vi "RGB to Color I2C.vi"(6 "B":u8, 7 "G":u8, 8 "R":u8) -> (0 "LEDout":i32[](array[numeric]), 1 "Blue Color":i32[](array[numeric]), 2 "Green Color":i32[](array[numeric]), 3 "Red Color":i32[](array[numeric]), 4 "Color":u32(colorbox))   [LabVIEW 2012]
doc: "Converts a red, green, and blue value from 0 to 255 to the corresponding RGB color."
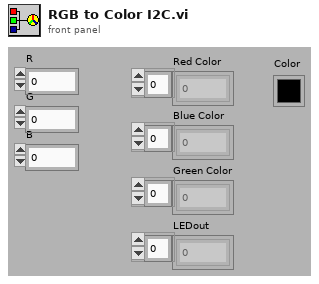
[diagram p1: front panel]
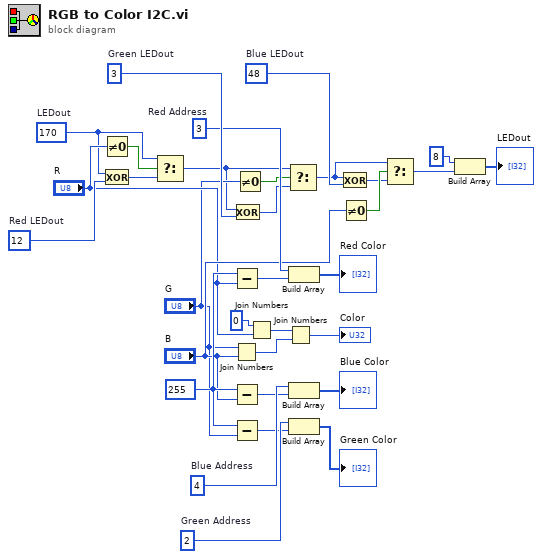
[diagram p0: block diagram]
diagram:
  w14 = 170  # LEDout
  w22 = 4  # Blue Address
  w16 = 2  # Green Address
  w24 = 3  # Red Address
  w25 = 48  # Blue LEDout
  w26 = 3  # Green LEDout
  w27 = 12  # Red LEDout
  w32 = 255
  n1 = Not Equal To 0?(x="R") -> (x != 0?=w15:bool)
  n2 = Exclusive Or(1:w27, 2:w14) -> (0:w13:i32)
  n3 = Select(t=w14, s=w15, f=w13) -> (s? t:f=w11:i32)
  n4 = Subtract(x=w32, y="R") -> (x-y=w3:i32)
  n5 = Join Numbers(hi="G", lo="B") -> ((hi.lo)=w29:u16)
  n6 = Subtract(x=w32, y="B") -> (x-y=w1:i32)
  n7 = Subtract(x=w32, y="G") -> (x-y=w2:i32)
  n8 = Exclusive Or(1:w26, 2:w11) -> (0:w10:i32)
  n9 = Not Equal To 0?(x="G") -> (x != 0?=w12:bool)
  n10 = Join Numbers(hi=u8 0, lo="R") -> ((hi.lo)=w30:u16)
  n11 = Join Numbers(hi=w30, lo=w29) -> ((hi.lo)=→"Color":u32)
  n12 = Select(t=w11, s=w12, f=w10) -> (s? t:f=w4:i32)
  n13 = Build Array(w24, w3) -> (→"Red Color":i32[])
  n14 = Build Array(w22, w1) -> (→"Blue Color":i32[])
  n15 = Build Array(w16, w2) -> (→"Green Color":i32[])
  n16 = Exclusive Or(1:w25, 2:w4) -> (0:w8:i32)
  n17 = Not Equal To 0?(x="B") -> (x != 0?=w9:bool)
  n18 = Select(t=w4, s=w9, f=w8) -> (s? t:f=w6:i32)
  n19 = Build Array(u8 8 ("element"), w6) -> (→"LEDout":i32[])
